vi "Connect to PPT Window.vi"(8 "error in (no error)":errorcluster, 9 "Index":i32, 11 "Application refnum":refnum<k7>) -> (0 "error out":errorcluster, 2 "Presentation refnum out":refnum<k7>, 3 "Application refnum out":refnum<k7>)   [LabVIEW 2018, in "lpptx.lvlib"]
uses:
  lpptx.lvlib
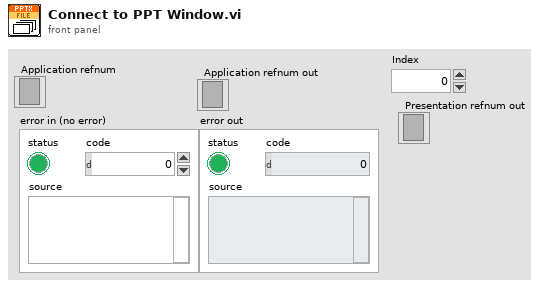
[diagram p1: front panel]
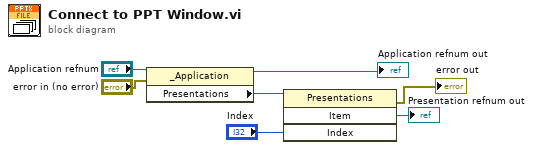
[diagram p0: block diagram]
diagram:
  n1 = property class="_Application"(reference="Application refnum", error in="error in (no error)") -> (reference out=→"Application refnum out":refnum<k7>, "Presentations"=w5:refnum<k7>)  [unwired: 1 out]
  n2 = invoke class="Presentations" method="Item"(reference=w5, "Index"="Index") -> (error out=→"error out":errorcluster, "Item"=→"Presentation refnum out":refnum<k7>)  [unwired: 2 in, 2 out]
